vi "Pre Test Case Reset.vi"(11 "LUnit Test Case In":refnum<class "LUnit Test Case.lvclass">) -> (3 "LUnit Test Case Out":refnum<class "LUnit Test Case.lvclass">)   [LabVIEW 2020, in "LUnit Test Case.lvclass"]
uses:
  LUnit Test Case.lvclass
  Result Classes/Test Case Result/Test Case Result.lvclass
  LUnit Test Case.lvclass/LUnit Test Case.ctl
  Result Classes/Method Result/Method Result.lvclass/Method Result.ctl
  Result Classes/Test Case Result/Test Case Result.lvclass/Test Case Result.ctl
  Public/Accessors/Read Enabled Test Methods.vi
  Private/SubVIs/Read Test Case Name.vi
  Result Classes/Test Case Result/Community/Preallocate Method Results.vi
  Result Classes/Method Result/Community/Accessors/Write Test Method Name.vi
  Result Classes/Method Result/Community/Accessors/Write Test Case.vi
  Result Classes/Method Result/Method Result.lvclass
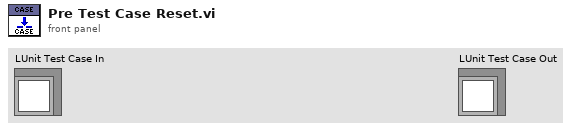
[diagram p1: front panel]
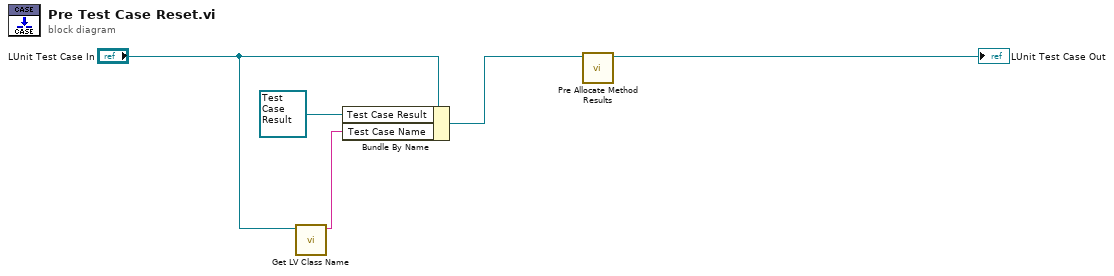
[diagram p0: block diagram]
diagram:
  n1 = call <vilib>:"Get LV Class Name.vi"("object"="LUnit Test Case In") -> ("class name"=w4:string)  [unwired: 9 in, 1 out]
  n2 = Bundle By Name(cluster="LUnit Test Case In", "Test Case Result"=refnum<class "Test Case Result.lvclass"> refnum, "Test Case Name"=w4) -> (w2:refnum<class "LUnit Test Case.lvclass">)
  n3 = call "Pre Allocate Method Results.vi"("LUnit Test Case In"=w2) -> ("LUnit Test Case Out"=→"LUnit Test Case Out":refnum<class "LUnit Test Case.lvclass">)  [unwired: 10 in]
